vi "Final_Implementation.vi"() -> ()   [LabVIEW 2016]
panel:
  in  "stop":bool
  out "frequency":dbl
  out "Waveform Chart":dynamicdata(graph)
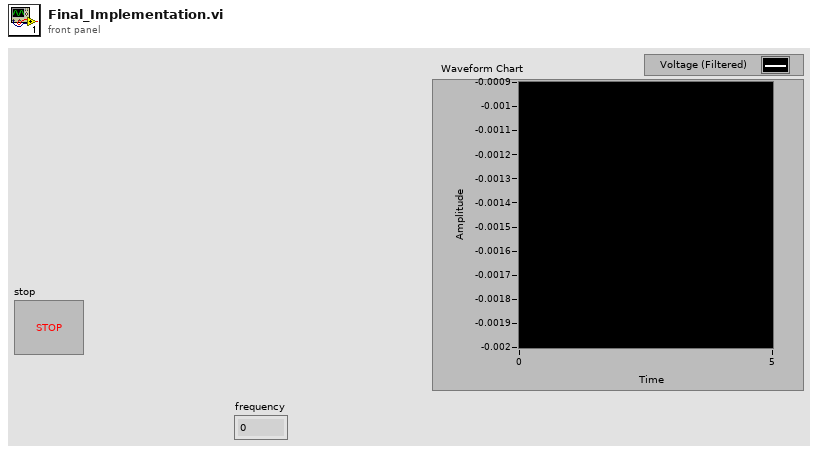
[diagram p1: front panel]
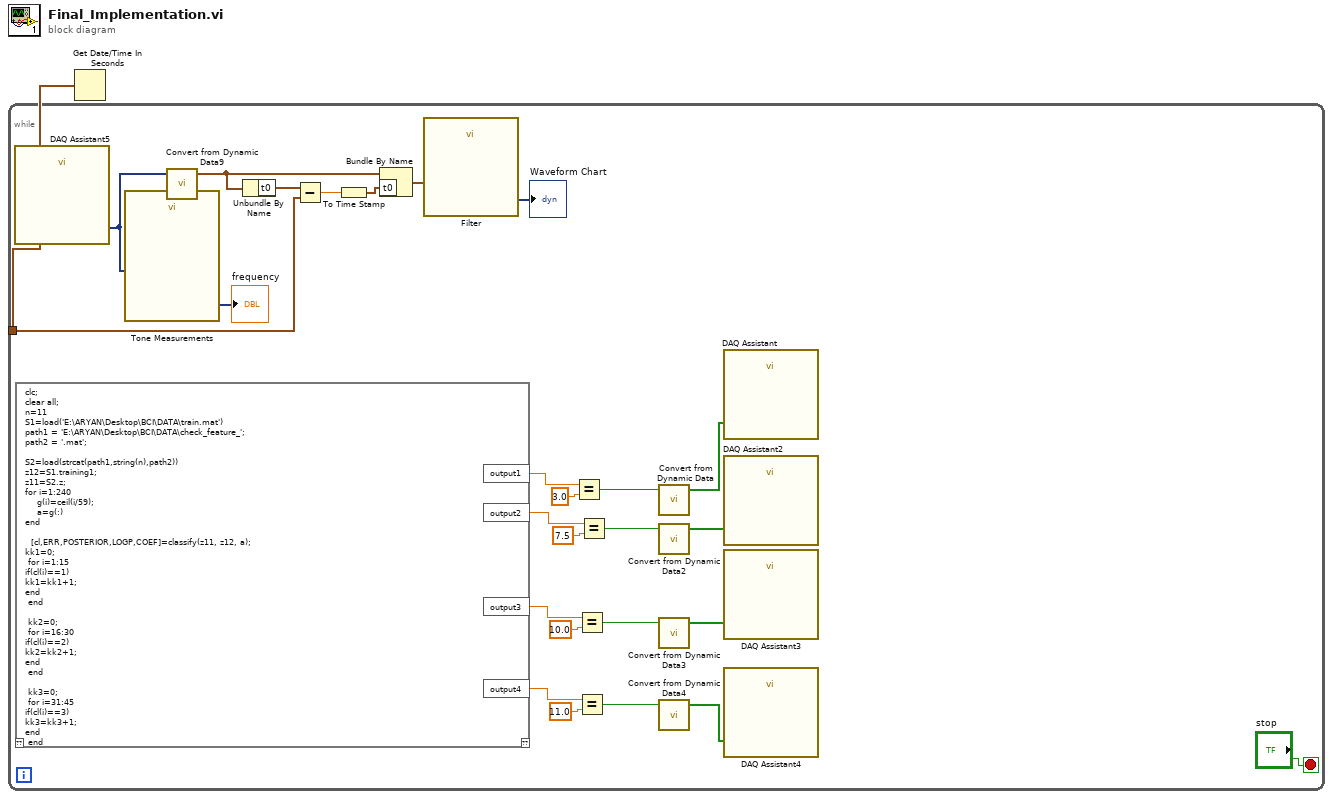
[diagram p0: block diagram]
diagram:
  n1 = Get Date/Time In Seconds() -> (seconds since 1Jan1904=w1:timestamp)
  n2 = while {
    tunnel: w1 -> [w26]
    stop <- "stop" stop-if-true
    n3 = call "DAQ Assistant5"() -> ("data"=w24:dynamicdata)  [unwired: 16 in, 3 out]
    n4 = script code="clc;\nclear all;\nn=11\nS1=load('E:\\ARYAN\\Desktop\\BCI\\DATA\\train.mat')\npath1 = 'E:\\ARYAN\\Desktop\\BCI\\DATA\\check_feature_';\npath2 = '.mat';\n\nS2=load(strcat(path1,string(n),path2))\nz12=S1.training1;\nz11=S2.z;\nfor i=1:240\n    g(i)=ceil(i/59);\n    a=g(:)\nend\n\n  [cl,ERR,POSTERIOR,LOGP,COEF]=classify(z11, z12, a);\nkk1=0;\n for i=1:15\nif(cl(i)==1)\nkk1=kk1+1;\nend\n end\n\n kk2=0;\n for i=16:30\nif(cl(i)==2)\nkk2=kk2+1;\nend\n end\n\n kk3=0;\n for i=31:45\nif(cl(i)==3)\nkk3=kk3+1;\nend\n end\n\n kk4=0;\n for i=46:59\nif(cl(i)==4)\nkk4=kk4+1;\nend\n end\n\n\nfprintf('\\nthe accuracy of class 1 is %d',(kk1/15)*100);\nfprintf('\\nthe accuracy of class 2 is %d',(kk2/15)*100);\nfprintf('\\nthe accuracy of class 3 is %d',(kk3/15)*100);\nfprintf('\\nthe accuracy of class 4 is %d',(kk4/14)*100);\n\nclass=[kk1 kk2 kk3 kk4];\nfinal = max(class)\nindex = find(class==final,1)\noutput1 = 0\noutput2 = 0\noutput3 = 0\noutput4 = 0\nif index == 1\noutput1 = 3\nelseif index == 2\noutput2 = 7.5\nelseif index == 3\noutput3 = 10\nelse\noutput4 = 11\nend"() -> ("output1"=w3:dbl, "output2"=w4:dbl, "output3"=w5:dbl, "output4"=w6:dbl)  [unwired: 1 in, 1 out]
    n5 = call "Tone Measurements"("Signals"=w24) -> ("Frequency"=→"frequency":dynamicdata)  [unwired: 8 in, 2 out]
    n6 = call "Convert from Dynamic Data9"("Dynamic Data Type"=w24) -> ("Waveform"=w21:waveform(dbl))  [unwired: 3 in]
    n7 = Unbundle By Name(w21) -> ("t0"=w23:timestamp)
    n8 = Subtract(x=w23, y=w26) -> (x-y=w25:dbl)
    n9 = To Time Stamp(1:w25) -> (0:w22:timestamp)
    n10 = Bundle By Name(cluster=w21, "t0"=w22) -> (w20:waveform(dbl))
    n11 = call "Filter"("Signal"=w20) -> ("Filtered Signal"=→"Waveform Chart":dynamicdata)  [unwired: 9 in, 1 out]
    n12 = Equal?(x=w3, y=3.0) -> (x = y?=w11:bool)
    n13 = Equal?(x=w5, y=10.0) -> (x = y?=w14:bool)
    n14 = Equal?(x=w6, y=11.0) -> (x = y?=w13:bool)
    n15 = Equal?(x=w4, y=7.5) -> (x = y?=w12:bool)
    n16 = call "Convert from Dynamic Data"("Dynamic Data Type"=w11) -> ("Array"=w15:bool[])  [unwired: 3 in]
    n17 = call "Convert from Dynamic Data2"("Dynamic Data Type"=w12) -> ("Array"=w16:bool[])  [unwired: 3 in]
    n18 = call "Convert from Dynamic Data3"("Dynamic Data Type"=w14) -> ("Array"=w17:bool[])  [unwired: 3 in]
    n19 = call "Convert from Dynamic Data4"("Dynamic Data Type"=w13) -> ("Array"=w18:bool[])  [unwired: 3 in]
    n20 = call "DAQ Assistant"("data"=w15) -> ()  [unwired: 17 in, 2 out]
    n21 = call "DAQ Assistant2"("data"=w16) -> ()  [unwired: 17 in, 2 out]
    n22 = call "DAQ Assistant3"("data"=w17) -> ()  [unwired: 17 in, 2 out]
    n23 = call "DAQ Assistant4"("data"=w18) -> ()  [unwired: 17 in, 2 out]
  }
